vi "WFM - XYSCAN.vi"(5 "Sampling rate":dbl=128000.0 format="%#_13g", 7 "Fast axis frequency":dbl=100.0, 8 "error in (no error)":errorcluster, 10 "Special coordinates (um)":T1, 11 "Frame Properties":T2={"Height (um)"=50.0, "Width (um)"=50.0, "Y Position (um)"=0.0, "X Position (um)"=0.0, "Y Resolution"=512.0}) -> (0 "error out":errorcluster, 3 "appended array":waveform(dbl)[](array[waveform]))   [LabVIEW 2017]
uses:
  <vilib>/measure/NI_MABase.lvlib
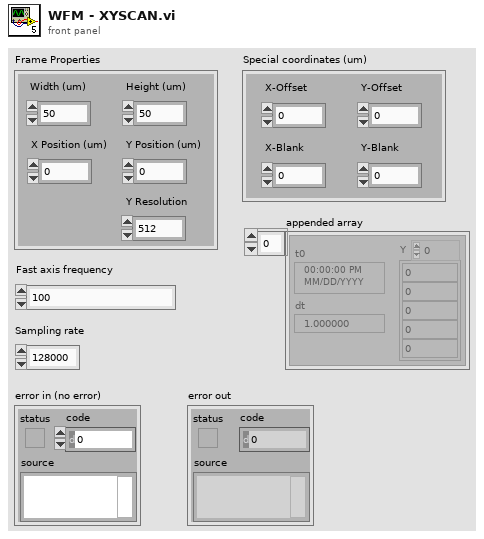
[diagram p1: front panel]
types:
  T1 = cluster{"Y-Offset":dbl, "X-Offset":dbl, "Y-Blank":dbl, "X-Blank":dbl}
  T2 = cluster{"Height (um)":dbl, "Width (um)":dbl, "Y Position (um)":dbl, "X Position (um)":dbl, "Y Resolution":dbl}
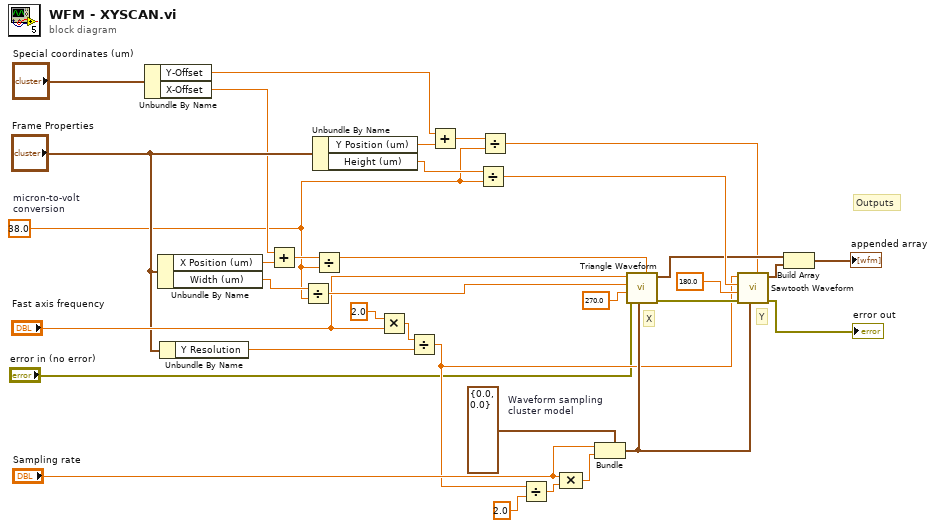
[diagram p0: block diagram]
diagram:
  w4 = 38.0  # micron-to-volt  conversion
  w20 = cluster{"Fs":dbl, "#s":dbl} {"Fs"=0.0, "#s"=0.0}  # Waveform sampling  cluster model
  # "Outputs"
  # "Y"
  # "X"
  n1 = Unbundle By Name("Special coordinates (um)") -> ("Y-Offset"=w10:dbl, "X-Offset"=w8:dbl)
  n2 = Unbundle By Name("Frame Properties") -> ("X Position (um)"=w7:dbl, "Width (um)"=w33:dbl)
  n3 = Unbundle By Name("Frame Properties") -> ("Y Resolution"=w14:dbl)
  n4 = Add(x=w8, y=w7) -> (x+y=w5:dbl)
  n5 = Divide(x=w33, y=w4) -> (x/y=w30:dbl)
  n6 = Unbundle By Name("Frame Properties") -> ("Y Position (um)"=w11:dbl, "Height (um)"=w32:dbl)
  n7 = Divide(x=w5, y=w4) -> (x/y=w6:dbl)
  n8 = Multiply(x=2.0 ("y"), y="Fast axis frequency") -> (x*y=w25:dbl)
  n9 = Divide(x=w25, y=w14) -> (x/y=w17:dbl)
  n10 = Add(x=w10, y=w11) -> (x+y=w9:dbl)
  n11 = Divide(x=w32, y=w4) -> (x/y=w31:dbl)
  n12 = Divide(x=w9, y=w4) -> (x/y=w1:dbl)
  n13 = Divide(x=w17, y=2.0) -> (x/y=w21:dbl)
  n14 = Compound Arithmetic op=MULTIPLY("Sampling rate", w21) -> (w23:dbl)
  n15 = Bundle(cluster=w20, "Fs"="Sampling rate", "#s"=w23) -> (w18:cluster{"Fs":dbl, "#s":dbl})
  n16 = call <vilib>:"Triangle Waveform.vi"("offset"=w6, "sampling info"=w18, "error in (no error)"="error in (no error)", "phase"=270.0, "amplitude"=w30, "frequency"="Fast axis frequency") -> ("error out"=w34:errorcluster, "signal out"=w13:waveform(dbl))  [unwired: 4 in]
  n17 = call <vilib>:"Sawtooth Waveform.vi"("offset"=w1, "sampling info"=w18, "error in (no error)"=w34, "phase"=180.0, "amplitude"=w31, "frequency"=w17) -> ("error out"=→"error out":errorcluster, "signal out"=w24:waveform(dbl))  [unwired: 4 in]
  n18 = Build Array(w13, w24) -> (→"appended array":waveform(dbl)[])
